vi "Rearrange Array 1D DBL.vi"(4 "Index Map":i32[][](array[numeric]), 6 "Array":dbl[](array[numeric])) -> (2 "Rearranged Array":dbl[](array[numeric]))   [LabVIEW 2013]
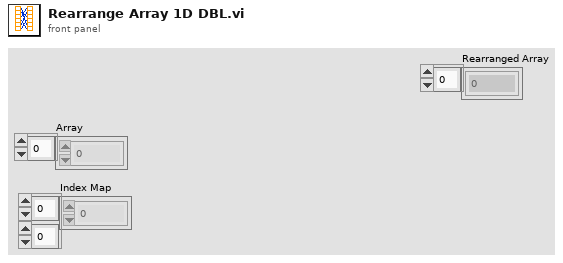
[diagram p1: front panel]
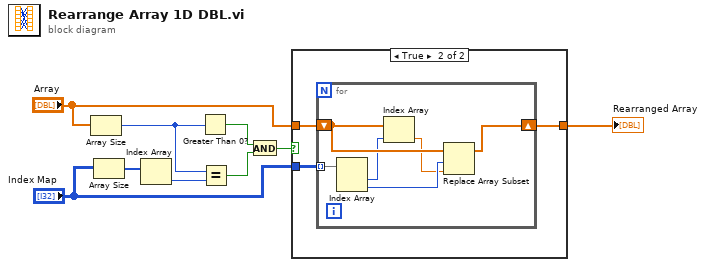
[diagram p0: block diagram]
diagram:
  n1 = Array Size(array="Array") -> (size(s)=w1:i32)
  n2 = Array Size(array="Index Map") -> (size(s)=w8:i32[])
  n3 = Index Array(array=w8) -> (element=w6:i32)  [unwired: 1 in]
  n4 = Greater Than 0?(x=w1) -> (x > 0?=w7:bool)
  n5 = Equal?(x=w1, y=w6) -> (x = y?=w4:bool)
  n6 = And(x=w7, y=w4) -> (x .and. y?=w5:bool)
  n7 = case shown="True" w5 {
    tunnel: "Index Map" -> [_ w13]
    tunnel: "Array" -> [w10 w12]
    tunnel: [w10 w11] -> w9
    frame False {
    }
    frame True {
      n8 = for {
        tunnel: w13 -> [w19] mode=indexing
        shift-right: [w14] -> w11
        shift-left: w12 -> [w18]
        n9 = Index Array(array=w19) -> (element #1=w17:i32, element #2=w16:i32)  [unwired: 2 in]
        n10 = Index Array(array=w18, index=w17) -> (element=w15:dbl)
        n11 = Replace Array Subset(array=w18, new element=w15, index=w16) -> (w14:dbl[])
      }
    }
  }
  "Rearranged Array" <- w9
